vi "Read Configure acceptance limits.vi"(8 "error in":errorcluster, 11 "数组 2":T3(array[ring])=[enum."VHEATFUSENOLOADMIN", enum."VHEATFUSELOADMAX", enum."VOVERRIDEDIODEMIN", enum."TDIFFMAX", enum."MEASFREQMAX", enum."MEASFREQMIN", enum."VOVER", enum."VMIDDLE", enum."VUNDER", enum."VNORESET", enum."VRESET", enum."WAITPING", enum."LRFID", enum."RFIDUID", enum."EXTEESIZE", enum."LCUTYPE", enum."LCUSUBTYPE", enum."TEVN", enum."BOOTVER", enum."APPVER", enum."ISLEEPMAX", enum."TSLEEP", enum."APPWAIT", enum."DBWAIT"]) -> (0 "error out":errorcluster, 1 "test path":T1, 2 "Product serial number":T2={"serial number"="", "Part number"="4821683", "Revision letter "="01", "Revision counter"="000", "Manufature"="005", "Year Week"=""}, 3 "acceptance Limits":T4, 4 "Write manufature data and test program":path, 5 "file path":path, 7 "number":i32)   [LabVIEW 2009]
uses:
  Global/Global 1.vi
  <vilib>/Utility/config.llb/Read Key (String).vi
  <vilib>/Utility/config.llb/NI_LVConfig.lvlib
panel:
  # "Read configure acceptance limit and manufature"
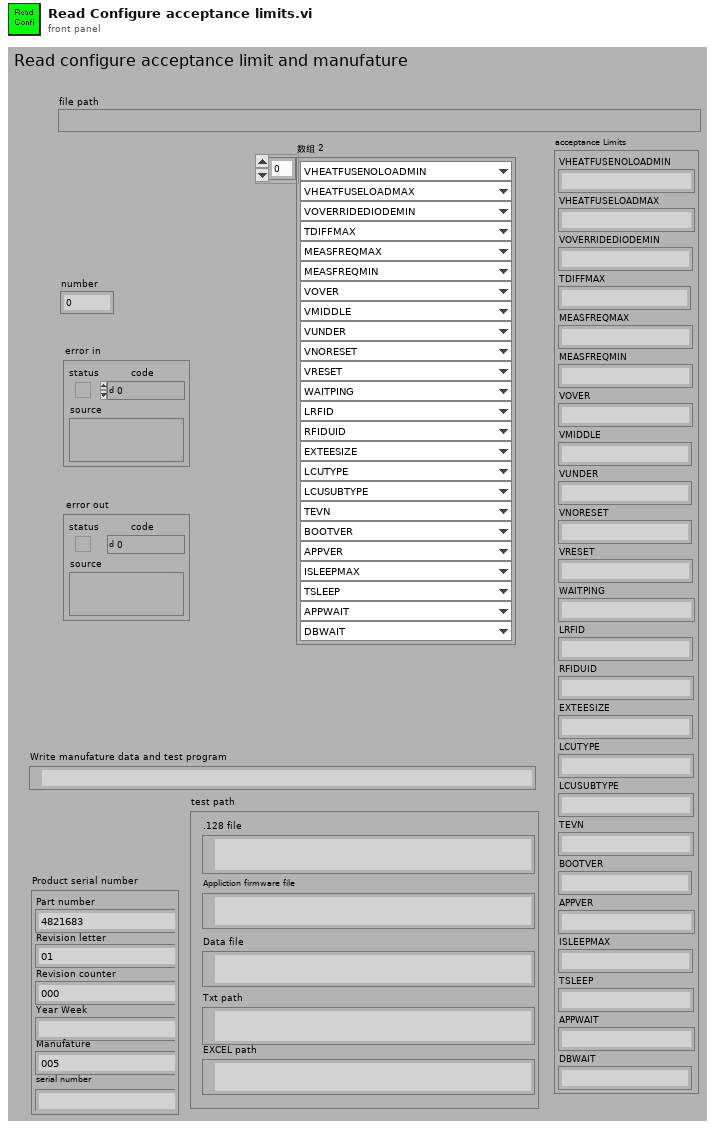
[diagram p1: front panel]
types:
  T1 = cluster{".128 file":path, "Appliction firmware file":path, "Data file":path, "Txt path":path, "EXCEL path":path}
  T2 = cluster{"serial number":string, "Part number":string, "Revision letter ":string, "Revision counter":string, "Manufature":string, "Year Week":string}
  T3 = enum16{"VHEATFUSENOLOADMIN", "VHEATFUSELOADMAX", "VOVERRIDEDIODEMIN", "TDIFFMAX", "MEASFREQMAX", "MEASFREQMIN", "VOVER", "VMIDDLE", "VUNDER", "VNORESET", "VRESET", "WAITPING", "LRFID", "RFIDUID", "EXTEESIZE", "LCUTYPE", "LCUSUBTYPE", "TEVN", "BOOTVER", "APPVER", "ISLEEPMAX", "TSLEEP", "APPWAIT", "DBWAIT"}[]
  T4 = cluster{"VHEATFUSENOLOADMIN":string, "VHEATFUSELOADMAX":string, "VOVERRIDEDIODEMIN":string, "TDIFFMAX":string, "MEASFREQMAX":string, "MEASFREQMIN":string, "VOVER":string, "VMIDDLE":string, "VUNDER":string, "VNORESET":string, "VRESET":string, "WAITPING":string, "LRFID":string, "RFIDUID":string, "EXTEESIZE":string, "LCUTYPE":string, "LCUSUBTYPE":string, "TEVN":string, "BOOTVER":string, "APPVER":string, "ISLEEPMAX":string, "TSLEEP":string, "APPWAIT":string, "DBWAIT":string}
  T5 = enum16{"Parr number", "Revision letter", "Revision counter", "Manufature", ".128 file", "Application firmware file", "Data file", "Txt path", "EXCLE path"}[]
  T6 = typedef "NI_LVConfig.lvlib/Config Data RefNum.ctl" = refnum<k1>
  T7 = cluster{"[0]":string, "[1]":string, "[2]":string, "[3]":string, "[4]":string, "[5]":string, "[6]":string, "[7]":string, "[8]":string, "[9]":string, "[10]":string, "[11]":string, "[12]":string, "[13]":string, "[14]":string, "[15]":string, "[16]":string, "[17]":string, "[18]":string, "[19]":string, "[20]":string, "[21]":string, "[22]":string, "[23]":string}
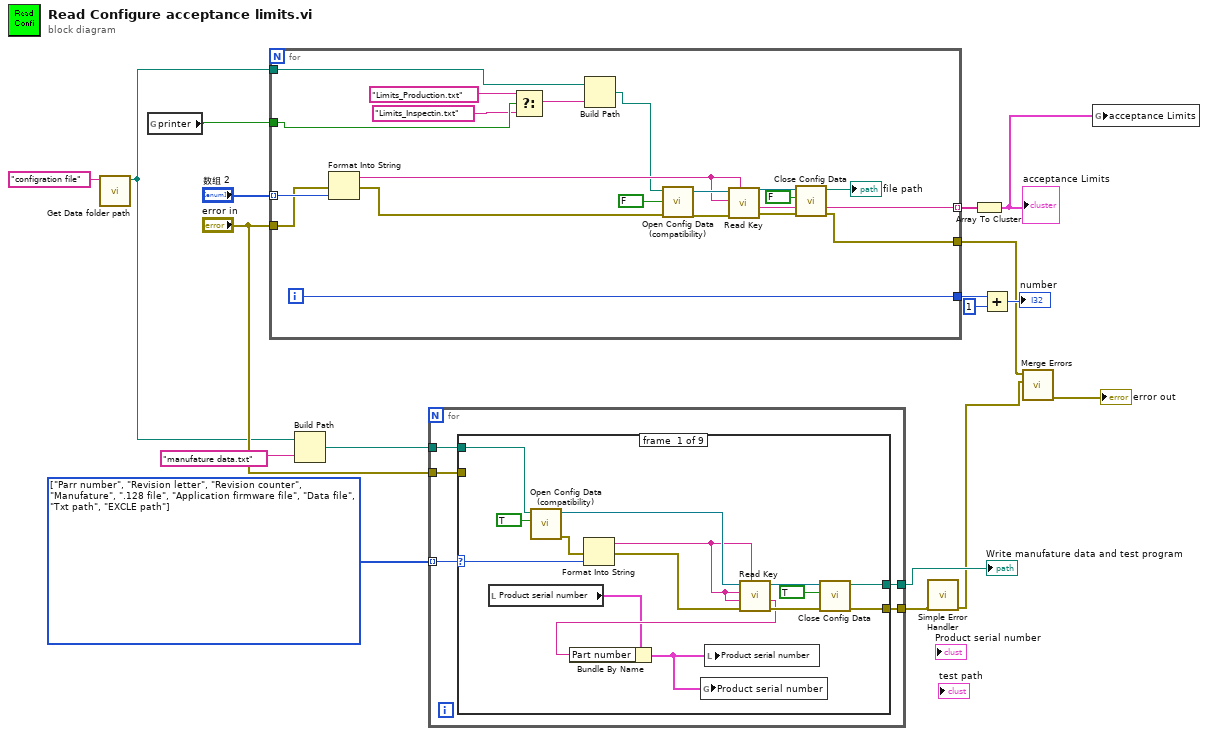
[diagram p0: block diagram]
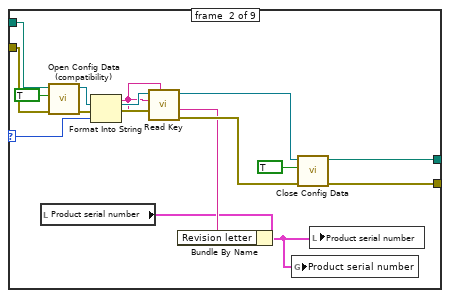
[diagram p2: hidden frame]
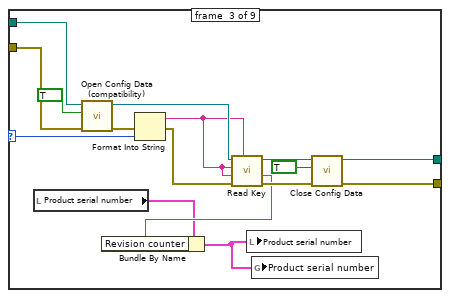
[diagram p3: hidden frame]
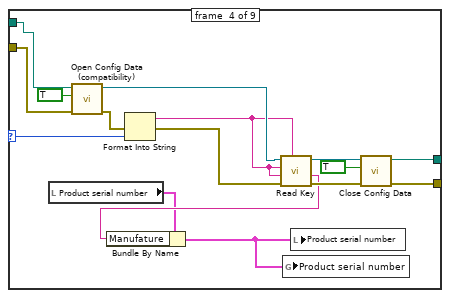
[diagram p4: hidden frame]
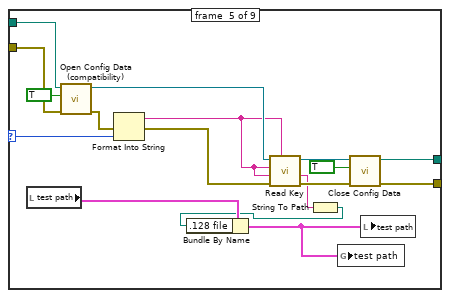
[diagram p5: hidden frame]
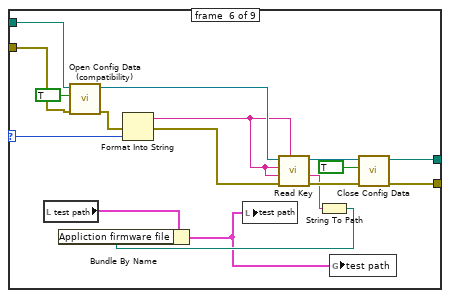
[diagram p6: hidden frame]
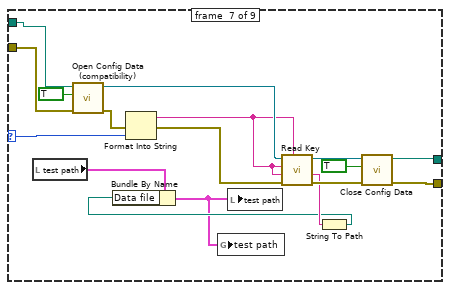
[diagram p7: hidden frame]
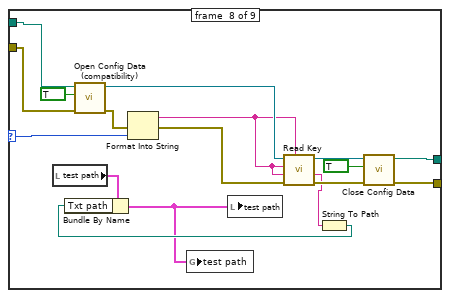
[diagram p8: hidden frame]
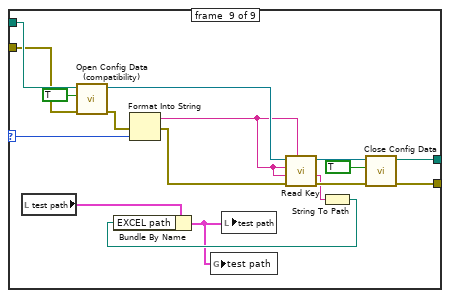
[diagram p9: hidden frame]
diagram:
  w13 = T5 [enum."Parr number", enum."Revision letter", enum."Revision counter", enum."Manufature", enum.".128 file", enum."Application firmware file", enum."Data file", enum."Txt path", enum."EXCLE path"] items=["Parr number", "Revision letter", "Revision counter", "Manufature", ".128 file", "Application firmware file", "Data file", "Txt path", "EXCLE path"]
  n1 = call "Get Data folder path.vi"("Data Path Name"="configration file") -> ("Data Path"=w2:path)  [unwired: 1 in, 9 out]
  n2 = global read "Global 1.vi" "printer"() -> (w1:bool)
  n3 = for {
    tunnel: [w31] -> w17 mode=indexing
    tunnel: "数组 2" -> [w30] mode=indexing
    tunnel: "error in" -> [w28]
    tunnel: [w26] -> w6
    tunnel: w1 -> [w24]
    tunnel: [w25] -> w16
    tunnel: w2 -> [w21]
    i -> [w25]
    n4 = Format Into String(error in=w28, w30) -> (resulting string=w29:string, error out=w27:errorcluster)  [unwired: 2 in]
    n5 = Select(t="Limits_Production.txt" ("名称或相对路径"), s=w24, f="Limits_Inspectin.txt" ("名称或相对路径")) -> (s? t:f=w20:string)
    n6 = Build Path(base path=w21, name or relative path=w20) -> (appended path=w19:path)
    n7 = call <vilib>:"Open Config Data (compatibility).vi"("error in (no error)"=w27, "create file if necessary (T)"=FALSE ("create file if necessary? (T)"), "configuration file path"=w19) -> ("error out"=w34:errorcluster, "refnum"=w35:T6)  [unwired: 6 in, 1 out]
    n8 = call-poly <vilib>:"Read Key.vi"("section"=w29, "error in (no error)"=w34, "key"=w29, "refnum"=w35) -> ("error out"=w36:errorcluster, "value"=w31:string, "refnum out"=w37:T6)  [unwired: 2 in, 3 out]
    n9 = call <vilib>:"Close Config Data.vi"("error in (no error)"=w36, "write file if changed (T)"=FALSE ("write configuration file? (T)"), "refnum"=w37) -> ("error out"=w26:errorcluster, "file path"=→"file path":path)  [unwired: 7 out]
  }
  n10 = Build Path(base path=w2, name or relative path="manufature data.txt" ("名称或相对路径")) -> (appended path=w11:path)
  n11 = for {
    tunnel: w13 -> [w43] mode=indexing
    tunnel: w11 -> [w42]
    tunnel: [w41] -> w12
    tunnel: "error in" -> [w40]
    tunnel: [w39] -> w9
    n12 = case shown="\"EXCLE path\"" w43 {
      selector: w43 -> [w49 w73 w83 w101 w118 w135 w152 w169 w186]
      tunnel: [w53 w67 w82 w99 w117 w133 w150 w167 w184] -> w41
      tunnel: w42 -> [w52 w71 w85 w100 w116 w134 w151 w168 w185]
      tunnel: w40 -> [_ w65 w80 w97 w114 w131 w148 w165 w182]
      tunnel: [w48 w64 w79 w96 w113 w130 w147 w164 w181] -> w39
      frame #0 {
        n13 = local read "Product serial number"() -> (w45:T2)
        n14 = call <vilib>:"Open Config Data (compatibility).vi"("create file if necessary (T)"=TRUE ("create file if necessary? (T)"), "configuration file path"=w52) -> ("error out"=w57:errorcluster, "refnum"=w50:T6)  [unwired: 7 in, 1 out]
        n15 = Format Into String(error in=w57, w49) -> (resulting string=w47:string, error out=w58:errorcluster)  [unwired: 2 in]
        n16 = call-poly <vilib>:"Read Key.vi"("section"=w47, "error in (no error)"=w58, "default value"=w47, "key"=w47, "refnum"=w50) -> ("error out"=w55:errorcluster, "value"=w46:string, "refnum out"=w54:T6)  [unwired: 1 in, 3 out]
        n17 = Bundle By Name(cluster=w45, "Part number"=w46) -> (w44:T2)
        n18 = global write "Global 1.vi" "Product serial number"(w44) -> ()
        n19 = local write "Product serial number"(w44) -> ()
        n20 = call <vilib>:"Close Config Data.vi"("error in (no error)"=w55, "write file if changed (T)"=TRUE ("write configuration file? (T)"), "refnum"=w54) -> ("error out"=w53:errorcluster, "file path"=w48:path)  [unwired: 7 out]
      }
      frame #1 {
        n21 = local read "Product serial number"() -> (w60:T2)
        n22 = call <vilib>:"Open Config Data (compatibility).vi"("error in (no error)"=w65, "create file if necessary (T)"=TRUE ("create file if necessary? (T)"), "configuration file path"=w71) -> ("error out"=w72:errorcluster, "refnum"=w66:T6)  [unwired: 6 in, 1 out]
        n23 = Format Into String(error in=w72, w73) -> (resulting string=w62:string, error out=w74:errorcluster)  [unwired: 2 in]
        n24 = call-poly <vilib>:"Read Key.vi"("section"=w62, "error in (no error)"=w74, "default value"=w62, "key"=w62, "refnum"=w66) -> ("error out"=w69:errorcluster, "value"=w61:string, "refnum out"=w68:T6)  [unwired: 1 in, 3 out]
        n25 = Bundle By Name(cluster=w60, "Revision letter"=w61) -> (w59:T2)
        n26 = global write "Global 1.vi" "Product serial number"(w59) -> ()
        n27 = call <vilib>:"Close Config Data.vi"("error in (no error)"=w69, "write file if changed (T)"=TRUE ("write configuration file? (T)"), "refnum"=w68) -> ("error out"=w67:errorcluster, "file path"=w64:path)  [unwired: 7 out]
        n28 = local write "Product serial number"(w59) -> ()
      }
      frame #2 {
        n29 = local read "Product serial number"() -> (w76:T2)
        n30 = call <vilib>:"Open Config Data (compatibility).vi"("error in (no error)"=w80, "create file if necessary (T)"=TRUE ("create file if necessary? (T)"), "configuration file path"=w85) -> ("error out"=w89:errorcluster, "refnum"=w81:T6)  [unwired: 6 in, 1 out]
        n31 = Format Into String(error in=w89, w83) -> (resulting string=w78:string, error out=w90:errorcluster)  [unwired: 2 in]
        n32 = call-poly <vilib>:"Read Key.vi"("section"=w78, "error in (no error)"=w90, "default value"=w78, "key"=w78, "refnum"=w81) -> ("error out"=w87:errorcluster, "value"=w77:string, "refnum out"=w86:T6)  [unwired: 1 in, 3 out]
        n33 = Bundle By Name(cluster=w76, "Revision counter"=w77) -> (w75:T2)
        n34 = local write "Product serial number"(w75) -> ()
        n35 = global write "Global 1.vi" "Product serial number"(w75) -> ()
        n36 = call <vilib>:"Close Config Data.vi"("error in (no error)"=w87, "write file if changed (T)"=TRUE ("write configuration file? (T)"), "refnum"=w86) -> ("error out"=w82:errorcluster, "file path"=w79:path)  [unwired: 7 out]
      }
      frame #3 {
        n37 = local read "Product serial number"() -> (w92:T2)
        n38 = call <vilib>:"Open Config Data (compatibility).vi"("error in (no error)"=w97, "create file if necessary (T)"=TRUE ("create file if necessary? (T)"), "configuration file path"=w100) -> ("error out"=w105:errorcluster, "refnum"=w98:T6)  [unwired: 6 in, 1 out]
        n39 = Format Into String(error in=w105, w101) -> (resulting string=w94:string, error out=w106:errorcluster)  [unwired: 2 in]
        n40 = call-poly <vilib>:"Read Key.vi"("section"=w94, "error in (no error)"=w106, "default value"=w94, "key"=w94, "refnum"=w98) -> ("error out"=w103:errorcluster, "value"=w93:string, "refnum out"=w102:T6)  [unwired: 1 in, 3 out]
        n41 = Bundle By Name(cluster=w92, "Manufature"=w93) -> (w91:T2)
        n42 = global write "Global 1.vi" "Product serial number"(w91) -> ()
        n43 = local write "Product serial number"(w91) -> ()
        n44 = call <vilib>:"Close Config Data.vi"("error in (no error)"=w103, "write file if changed (T)"=TRUE ("write configuration file? (T)"), "refnum"=w102) -> ("error out"=w99:errorcluster, "file path"=w96:path)  [unwired: 7 out]
      }
      frame #4 {
        n45 = local read "test path"() -> (w109:T1)
        n46 = call <vilib>:"Open Config Data (compatibility).vi"("error in (no error)"=w114, "create file if necessary (T)"=TRUE ("create file if necessary? (T)"), "configuration file path"=w116) -> ("error out"=w122:errorcluster, "refnum"=w115:T6)  [unwired: 6 in, 1 out]
        n47 = Format Into String(error in=w122, w118) -> (resulting string=w111:string, error out=w123:errorcluster)  [unwired: 2 in]
        n48 = call-poly <vilib>:"Read Key.vi"("section"=w111, "error in (no error)"=w123, "default value"=w111, "key"=w111, "refnum"=w115) -> ("error out"=w120:errorcluster, "value"=w110:string, "refnum out"=w119:T6)  [unwired: 1 in, 3 out]
        n49 = String To Path(string=w110) -> (path=w108:path)
        n50 = Bundle By Name(cluster=w109, ".128 file"=w108) -> (w107:T1)
        n51 = global write "Global 1.vi" "test path"(w107) -> ()
        n52 = call <vilib>:"Close Config Data.vi"("error in (no error)"=w120, "write file if changed (T)"=TRUE ("write configuration file? (T)"), "refnum"=w119) -> ("error out"=w117:errorcluster, "file path"=w113:path)  [unwired: 7 out]
        n53 = local write "test path"(w107) -> ()
      }
      frame #5 {
        n54 = local read "test path"() -> (w126:T1)
        n55 = call <vilib>:"Open Config Data (compatibility).vi"("error in (no error)"=w131, "create file if necessary (T)"=TRUE ("create file if necessary? (T)"), "configuration file path"=w134) -> ("error out"=w139:errorcluster, "refnum"=w132:T6)  [unwired: 6 in, 1 out]
        n56 = Format Into String(error in=w139, w135) -> (resulting string=w128:string, error out=w140:errorcluster)  [unwired: 2 in]
        n57 = call-poly <vilib>:"Read Key.vi"("section"=w128, "error in (no error)"=w140, "default value"=w128, "key"=w128, "refnum"=w132) -> ("error out"=w137:errorcluster, "value"=w127:string, "refnum out"=w136:T6)  [unwired: 1 in, 3 out]
        n58 = String To Path(string=w127) -> (path=w125:path)
        n59 = Bundle By Name(cluster=w126, "Appliction firmware file"=w125) -> (w124:T1)
        n60 = local write "test path"(w124) -> ()
        n61 = global write "Global 1.vi" "test path"(w124) -> ()
        n62 = call <vilib>:"Close Config Data.vi"("error in (no error)"=w137, "write file if changed (T)"=TRUE ("write configuration file? (T)"), "refnum"=w136) -> ("error out"=w133:errorcluster, "file path"=w130:path)  [unwired: 7 out]
      }
      frame #6 {
        n63 = local read "test path"() -> (w143:T1)
        n64 = call <vilib>:"Open Config Data (compatibility).vi"("error in (no error)"=w148, "create file if necessary (T)"=TRUE ("create file if necessary? (T)"), "configuration file path"=w151) -> ("error out"=w156:errorcluster, "refnum"=w149:T6)  [unwired: 6 in, 1 out]
        n65 = Format Into String(error in=w156, w152) -> (resulting string=w145:string, error out=w157:errorcluster)  [unwired: 2 in]
        n66 = call-poly <vilib>:"Read Key.vi"("section"=w145, "error in (no error)"=w157, "default value"=w145, "key"=w145, "refnum"=w149) -> ("error out"=w154:errorcluster, "value"=w144:string, "refnum out"=w153:T6)  [unwired: 1 in, 3 out]
        n67 = String To Path(string=w144) -> (path=w142:path)
        n68 = Bundle By Name(cluster=w143, "Data file"=w142) -> (w141:T1)
        n69 = global write "Global 1.vi" "test path"(w141) -> ()
        n70 = local write "test path"(w141) -> ()
        n71 = call <vilib>:"Close Config Data.vi"("error in (no error)"=w154, "write file if changed (T)"=TRUE ("write configuration file? (T)"), "refnum"=w153) -> ("error out"=w150:errorcluster, "file path"=w147:path)  [unwired: 7 out]
      }
      frame #7 {
        n72 = local read "test path"() -> (w160:T1)
        n73 = call <vilib>:"Open Config Data (compatibility).vi"("error in (no error)"=w165, "create file if necessary (T)"=TRUE ("create file if necessary? (T)"), "configuration file path"=w168) -> ("error out"=w173:errorcluster, "refnum"=w166:T6)  [unwired: 6 in, 1 out]
        n74 = Format Into String(error in=w173, w169) -> (resulting string=w162:string, error out=w174:errorcluster)  [unwired: 2 in]
        n75 = call-poly <vilib>:"Read Key.vi"("section"=w162, "error in (no error)"=w174, "default value"=w162, "key"=w162, "refnum"=w166) -> ("error out"=w171:errorcluster, "value"=w161:string, "refnum out"=w170:T6)  [unwired: 1 in, 3 out]
        n76 = String To Path(string=w161) -> (path=w159:path)
        n77 = Bundle By Name(cluster=w160, "Txt path"=w159) -> (w158:T1)
        n78 = global write "Global 1.vi" "test path"(w158) -> ()
        n79 = local write "test path"(w158) -> ()
        n80 = call <vilib>:"Close Config Data.vi"("error in (no error)"=w171, "write file if changed (T)"=TRUE ("write configuration file? (T)"), "refnum"=w170) -> ("error out"=w167:errorcluster, "file path"=w164:path)  [unwired: 7 out]
      }
      frame #8 {
        n81 = local read "test path"() -> (w177:T1)
        n82 = call <vilib>:"Open Config Data (compatibility).vi"("error in (no error)"=w182, "create file if necessary (T)"=TRUE ("create file if necessary? (T)"), "configuration file path"=w185) -> ("error out"=w190:errorcluster, "refnum"=w183:T6)  [unwired: 6 in, 1 out]
        n83 = Format Into String(error in=w190, w186) -> (resulting string=w179:string, error out=w191:errorcluster)  [unwired: 2 in]
        n84 = call-poly <vilib>:"Read Key.vi"("section"=w179, "error in (no error)"=w191, "default value"=w179, "key"=w179, "refnum"=w183) -> ("error out"=w188:errorcluster, "value"=w178:string, "refnum out"=w187:T6)  [unwired: 1 in, 3 out]
        n85 = String To Path(string=w178) -> (path=w176:path)
        n86 = Bundle By Name(cluster=w177, "EXCEL path"=w176) -> (w175:T1)
        n87 = global write "Global 1.vi" "test path"(w175) -> ()
        n88 = local write "test path"(w175) -> ()
        n89 = call <vilib>:"Close Config Data.vi"("error in (no error)"=w188, "write file if changed (T)"=TRUE ("write configuration file? (T)"), "refnum"=w187) -> ("error out"=w184:errorcluster, "file path"=w181:path)  [unwired: 7 out]
      }
    }
  }
  "Write manufature data and test program" <- w9
  n90 = call <vilib>:"Simple Error Handler.vi"("error in (no error)"=w12) -> ("error out"=w7:errorcluster)  [unwired: 1 in, 7 out]
  n91 = Array To Cluster(array=w17) -> (cluster=w4:T7)
  "acceptance Limits" <- w4
  n92 = Add(x=w16, y=1) -> (x+y=→"number":i32)
  n93 = call <vilib>:"Merge Errors.vi"("error in 2 (no error)"=w7, "error in 1 (no error)"=w6) -> ("error out"=→"error out":errorcluster)  [unwired: 2 in, 3 out]
  n94 = global write "Global 1.vi" "acceptance Limits"(w4) -> ()
